vi "Agilent 3352X Series Arbitrary Waveform Phase.vi"() -> ()   [LabVIEW 2020, in "AWG.lvlib"]
doc: "This example shows how to create then configure an phase of arbitrary waveform.\n\n<b>Note</b>:\nThis example is only available for 33600 series models."
uses:
  AWG.lvlib
  Instance           1 53Saved   Agilent 3352X Series Arbitrary Waveform Phase .vi
  Instance           2 53Saved   Agilent 3352X Series Arbitrary Waveform Phase .vi
  Agilent 3352X Series.lvlib
panel:
  in  "Sample Rate (40000 Sa/s)":dbl=40000.0
  in  "Phase Offset (0 Degree)":dbl
  in  "Units (0: Degree)":i32(ring) items=["Degree", "Radian", "Second", "Sample"]
  in  "Gain (0.1 Vpp)":dbl=0.1
  in  "Arbitrary Waveform Name":string="ARB1"
  in  "VISA resource name":refnum<visa-resource-name>
  # "(c) 2011-2015  National Instruments.  ALL RIGHTS RESERVED."
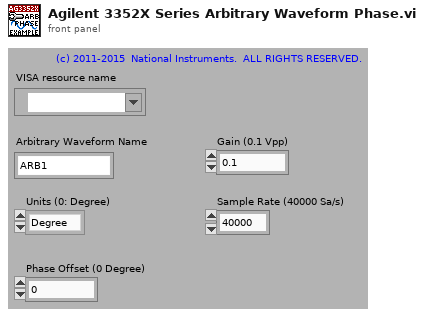
[diagram p1: front panel]
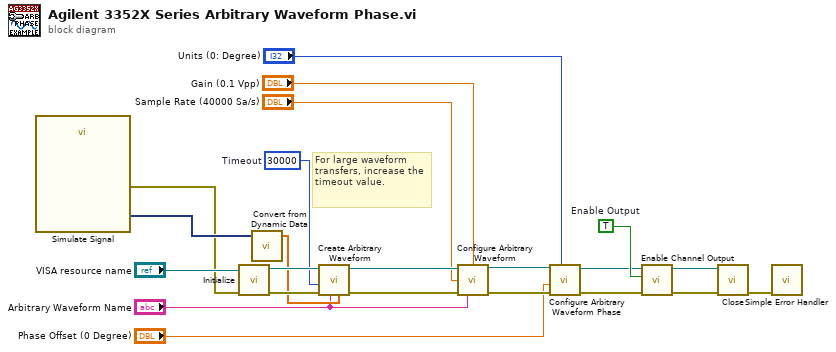
[diagram p0: block diagram]
diagram:
  w14 = TRUE  # Enable Output
  w8 = u32 30000  # Timeout
  # "For large waveform transfers, increase the timeout value."
  n1 = call "Simulate Signal"() -> ("Sine with Uniform Noise"=w22:dynamicdata, "error out"=w20:errorcluster)  [unwired: 8 in, 6 out]
  n2 = call "Initialize.vi"("error in (no error)"=w20, "VISA resource name"="VISA resource name") -> ("error out"=w16:errorcluster, "VISA resource name out"=w15:refnum<visa-resource-name>)  [unwired: 2 in, 6 out]
  n3 = call "Convert from Dynamic Data"("Dynamic Data Type"=w22) -> ("Array"=w10:dbl[])  [unwired: 3 out]
  n4 = call "Create Arbitrary Waveform.vi"("Arbitrary Waveform Data"=w10, "Arbitrary Waveform Name (ARB1)"="Arbitrary Waveform Name", "error in (no error)"=w16, "Timeout (10000 ms)"=w8, "VISA resource name"=w15) -> ("error out"=w12:errorcluster, "VISA resource name out"=w13:refnum<visa-resource-name>)  [unwired: 2 in, 3 out]
  n5 = call "Configure Arbitrary Waveform.vi"("VISA resource name"=w13, "Amplitude (0.1 Vpp)"="Gain (0.1 Vpp)", "Sample Rate (40000 Sa/s)"="Sample Rate (40000 Sa/s)", "error in (no error)"=w12, "Arbitrary Waveform (ARB1)"="Arbitrary Waveform Name") -> ("VISA resource name out"=w7:refnum<visa-resource-name>, "error out"=w6:errorcluster)  [unwired: 5 in, 4 out]
  n6 = call "Configure Arbitrary Waveform Phase.vi"("Units (0: Degree)"="Units (0: Degree)", "error in (no error)"=w6, "Phase Offset (0 Degree)"="Phase Offset (0 Degree)", "VISA resource name"=w7) -> ("error out"=w4:errorcluster, "VISA resource name out"=w5:refnum<visa-resource-name>)  [unwired: 1 in, 5 out]
  n7 = call "Enable Channel Output.vi"("error in (no error)"=w4, "Enable Output (T: Enable)"=w14, "VISA resource name"=w5) -> ("error out"=w18:errorcluster, "VISA resource name out"=w17:refnum<visa-resource-name>)  [unwired: 2 in, 5 out]
  n8 = call "Close.vi"("error in (no error)"=w18, "VISA resource name"=w17) -> ("error out"=w19:errorcluster)  [unwired: 9 out]
  n9 = call <vilib>:"Simple Error Handler.vi"("error in (no error)"=w19) -> ()  [unwired: 1 in, 8 out]
